vi "Variant to Class.vi"(8 "error in (no error)":errorcluster, 10 "Data in":variant, 11 "VI Analyzer Node in":refnum<class "VI Tester Node.lvclass">) -> (0 "error out":errorcluster, 2 "Data Out":variant, 3 "VI Analyzer Node out":refnum<class "VI Tester Node.lvclass">)   [LabVIEW 2014, in "VI Tester Node.lvclass"]
uses:
  VI Tester Node.lvclass
  Shared/Controls/VI Tester - STYP.ctl
  VI Tester Node.lvclass/VI Tester Node.ctl
  Classes/Build Job/Build Job.lvclass
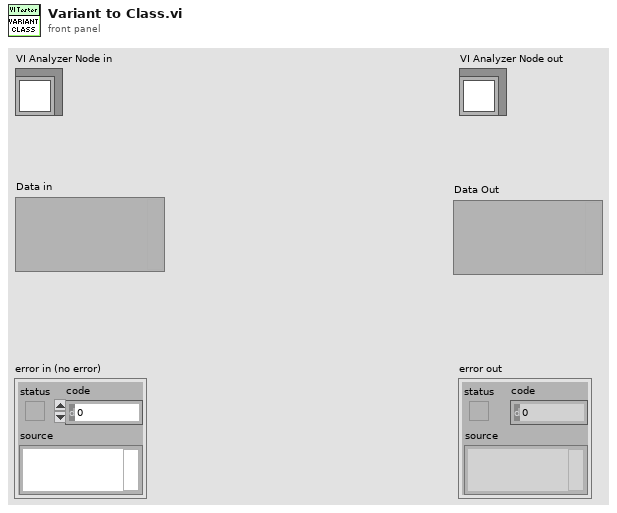
[diagram p1: front panel]
types:
  T1 = typedef "VI Tester - STYP.ctl" = cluster{"Executor_Number":string, "Workspace_Path":string, "Test Case":string}
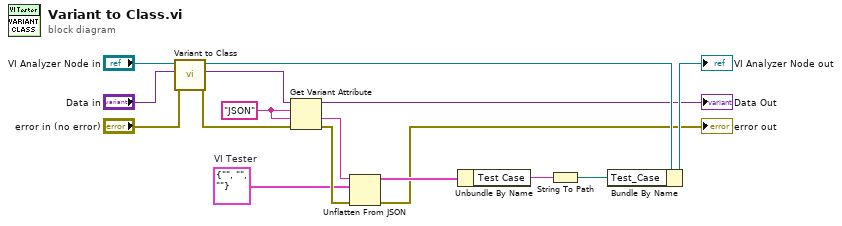
[diagram p0: block diagram]
diagram:
  w2 = T1 {"Executor_Number"="", "Workspace_Path"="", "Test Case"=""}  # VI Tester
  w14 = "JSON" ("name")
  n1 = call-parent "Variant to Class.vi"("error in (no error)"="error in (no error)", "Data in"="Data in", "Build Job in"="VI Analyzer Node in") -> ("error out"=w6:errorcluster, "Data Out"=w3:variant, "Build Job out"=w8:refnum<class "VI Tester Node.lvclass">)  [unwired: 6 in]
  n2 = Get Variant Attribute(Variant=w3, name=w14, default value (empty Variant)=w14, error in=w6) -> (duplicate Variant=→"Data Out":variant, value=w13:string, error out=w9:errorcluster)  [unwired: 1 out]
  n3 = Unflatten From JSON(JSON string=w13, type and defaults=w2, error in (no error)=w9) -> (value=w12:T1, error out=→"error out":errorcluster)  [unwired: 4 in]
  n4 = Unbundle By Name(w12) -> ("Test Case"=w11:string)
  n5 = String To Path(string=w11) -> (path=w10:path)
  n6 = Bundle By Name(cluster=w8, "Test_Case"=w10) -> (→"VI Analyzer Node out":refnum<class "VI Tester Node.lvclass">)
